vi "ObjectPool Pointer Test.vi"() -> ()   [LabVIEW 2016]
uses:
  Source/Submodules/Memory/Source/Classes/Internal/Memory.Pointer.Internal.lvclass
  C:/Git/Sourcetree/DSF/Source/Submodules/Memory/Source/Classes/Pointer/Memory.Pointer.lvclass
  Source/Submodules/Memory/Source/Classes/Pointer/Memory.Pointer.lvclass/Memory.Pointer.ctl
  Source/Engine/Classes/Pool/DSF.Engine.Memory.ObjectPool.lvclass/DSF.Engine.Memory.ObjectPool.ctl
  Source/Engine/Classes/Pool/DSF.Engine.Memory.ObjectPool.Bundle.lvclass/DSF.Engine.Memory.ObjectPool.Bundle.ctl
  Source/Submodules/Memory/Source/Classes/Pointer/Memory.Pointer.Write.Safe.0D.DBL.vi
  Source/Submodules/Memory/Source/Classes/Pointer/Memory.Pointer.Read.Safe.0D.DBL.vi
  Source/Submodules/Memory/Source/Classes/Pointer/Memory.Pointer.Write.Unsafe.0D.DBL.vi
  Source/Submodules/Memory/Source/Classes/Pointer/Memory.Pointer.Parameter Check.Null Pointer.vi
  Source/Submodules/Memory/Source/Classes/Pointer/Memory.Pointer.Parameter Check.Subset.vi
  Source/Engine/Classes/Pool/DSF.Engine.Memory.ObjectPool.Obtain Index.vi
  Source/Engine/Classes/Pool/DSF.Engine.Memory.ObjectPool.Get Object.vi
  Source/Engine/Classes/Pool/DSF.Engine.Memory.ObjectPool.Bundle.Create.vi
  Source/Submodules/Memory/Source/Classes/Pointer/Memory.Pointer.Read.Unsafe.0D.DBL.vi
  Source/Engine/Classes/Pool/DSF.Engine.Memory.ObjectPool.Bundle.Valid.vi
  Source/Engine/Classes/Pool/DSF.Engine.Memory.ObjectPool.Return Index.vi
  Source/Engine/Classes/Pool/DSF.Engine.Memory.ObjectPool.Bundle.Get Index.vi
  Source/Engine/Classes/Pool/DSF.Engine.Memory.ObjectPool.Set Object.vi
  Source/Submodules/Memory/Source/Classes/Pointer/Memory.Pointer.Get Address.vi
  Source/Submodules/Memory/Source/Classes/Pointer/Memory.Pointer.Errors.vi
  Source/Submodules/Memory/Source/Classes/Pointer/Memory.Pointer.Errors.Null Pointer.vi
  Source/Submodules/Memory/Source/Classes/Pointer/Memory.Pointer.Errors.Out of Bounds.vi
  Source/Submodules/Memory/Source/Classes/Pointer/Memory.Pointer.Get Size.vi
  Source/Engine/Classes/Pool/DSF.Engine.Memory.ObjectPool.Get Index FIFO.vi
  Source/Engine/Classes/Pool/DSF.Engine.Memory.ObjectPool.Bundle.Set Index.vi
  Source/Engine/Classes/Pool/DSF.Engine.Memory.ObjectPool.Bundle.Set Object.vi
  Source/Submodules/Memory/Source/Classes/Pointer/Memory.Pointer.Errors.Create Error.vi
  Source/Submodules/Memory/Source/Submodules/SEH/Source/VIs/Static Error Handling.Source Buffer.Write.String.vi
  Source/Submodules/Memory/Source/Classes/Pointer/Memory.Pointer.Errors.Write Pointer Size.vi
  Source/Submodules/Memory/Source/Submodules/SEH/Source/VIs/Static Error Handling.Source Buffer.Write.Numeric.Scalar.Base10.vi
  Source/Submodules/Memory/Source/Submodules/SEH/Source/VIs/Static Error Handling.Source Buffer.Write.Numeric.Scalar.Base10 (U64).vi
  Source/Submodules/Memory/Source/Submodules/SEH/Source/VIs/Static Error Handling.Error Cluster Constant.vi
  Source/Submodules/Memory/Source/Submodules/SEH/Source/VIs/Static Error Handling.Error Cluster Constant (256B).vi
  Source/Submodules/Memory/Source/Submodules/SEH/Source/VIs/Static Error Handling.Parameters.Status.Set.vi
  Source/Submodules/Memory/Source/Submodules/SEH/Source/VIs/Static Error Handling.Parameters.Code.Set.vi
  Source/Submodules/Memory/Source/Submodules/SEH/Source/VIs/Static Error Handling.Parameters.VI Source.Set.vi
  Source/Submodules/Memory/Source/Constants/Memory.Constants.vi
  Source/Submodules/Memory/Source/Constants/Memory.Constants.Library Name.vi
  Source/Submodules/Memory/Source/Classes/Pointer/Memory.Pointer.Errors.Get Info.vi
  Source/Submodules/Memory/Source/Classes/Internal/Memory.Pointer.Internal.Allocate.vi
  Source/Engine/Classes/Pool/DSF.Engine.Memory.ObjectPool.Bundle.lvclass
  Source/Engine/Classes/Pool/DSF.Engine.Memory.ObjectPool.lvclass
  Source/Submodules/Memory/Source/Classes/Pointer/Memory.Pointer.lvclass
panel:
  in  "value in":dbl=42.0
  out "value out":dbl
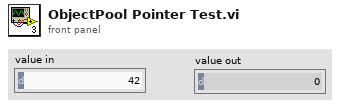
[diagram p1: front panel]
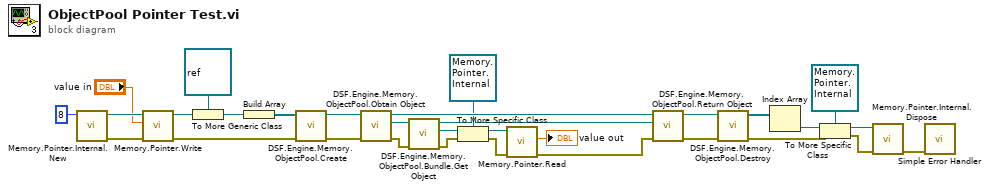
[diagram p0: block diagram]
diagram:
  n1 = call "Memory.Pointer.Internal.New.vi"("size"=u64 8) -> ("error out"=w24:errorcluster, "pointer"=w25:refnum<class "Memory.Pointer.Internal.lvclass">)  [unwired: 9 in]
  n2 = call-poly "Memory.Pointer.Write.vi"("error in (no error)"=w24, "value"="value in", "pointer in"=w25) -> ("error out"=w23:errorcluster, "pointer out"=w22:refnum<class "Memory.Pointer.Internal.lvclass">)  [unwired: 5 in, 2 out]
  n3 = To More Generic Class(target class=refnum<class> refnum ("LabVIEW Object"), reference=w22) -> (generic class reference=w20:refnum<class>)
  n4 = Build Array(w20) -> (w19:refnum<class>[])
  n5 = call "DSF.Engine.Memory.ObjectPool.Create.vi"("error in (no error)"=w23, "Objects"=w19) -> ("error out"=w28:errorcluster, "ObjectPool"=w31:refnum<class "DSF.Engine.Memory.ObjectPool.lvclass">)  [unwired: 8 in]
  n6 = call "DSF.Engine.Memory.ObjectPool.Obtain Object.vi"("error in (no error)"=w28, "ObjectPool in"=w31) -> ("error out"=w15:errorcluster, "ObjectPool Bundle"=w18:refnum<class "DSF.Engine.Memory.ObjectPool.Bundle.lvclass">, "ObjectPool out"=w30:refnum<class "DSF.Engine.Memory.ObjectPool.lvclass">)  [unwired: 6 in, 1 out]
  n7 = call "DSF.Engine.Memory.ObjectPool.Bundle.Get Object.vi"("error in (no error)"=w15, "ObjectPool Bundle in"=w18) -> ("error out"=w14:errorcluster, "Object"=w16:refnum<class>, "ObjectPool Bundle out"=w9:refnum<class "DSF.Engine.Memory.ObjectPool.Bundle.lvclass">)  [unwired: 7 in]
  n8 = To More Specific Class(target class=refnum<class "Memory.Pointer.Internal.lvclass"> refnum ("pointer out"), reference=w16, error in=w14) -> (specific class reference=w13:refnum<class "Memory.Pointer.Internal.lvclass">, error out=w12:errorcluster)
  n9 = call-poly "Memory.Pointer.Read.vi"("error in (no error)"=w12, "pointer in"=w13) -> ("error out"=w8:errorcluster, "value out"=→"value out":dbl)  [unwired: 6 in, 2 out]
  n10 = call "DSF.Engine.Memory.ObjectPool.Return Object.vi"("error in (no error)"=w8, "ObjectPool Bundle"=w9, "ObjectPool in"=w30) -> ("error out"=w27:errorcluster, "ObjectPool out"=w29:refnum<class "DSF.Engine.Memory.ObjectPool.lvclass">)  [unwired: 6 in, 1 out]
  n11 = call "DSF.Engine.Memory.ObjectPool.Destroy.vi"("error in (no error)"=w27, "ObjectPool"=w29) -> ("error out"=w4:errorcluster, "Objects"=w5:refnum<class>[])  [unwired: 8 in]
  n12 = Index Array(array=w5) -> (element=w6:refnum<class>)  [unwired: 1 in]
  n13 = To More Specific Class(target class=refnum<class "Memory.Pointer.Internal.lvclass"> refnum ("pointer out"), reference=w6, error in=w4) -> (specific class reference=w3:refnum<class "Memory.Pointer.Internal.lvclass">, error out=w2:errorcluster)
  n14 = call "Memory.Pointer.Internal.Dispose.vi"("error in (no error)"=w2, "pointer"=w3) -> ("error out"=w1:errorcluster)  [unwired: 9 in]
  n15 = call <vilib>:"Simple Error Handler.vi"("error in (no error)"=w1) -> ()  [unwired: 4 in, 5 out]
